vi "position_calculation.vi"(8 "bucket_angle":dbl, 9 "arm_angle":dbl, 10 "boom_angle":dbl) -> (2 "end_point":cluster{"x_axis":dbl, "z_axis":dbl})   [LabVIEW 2020]
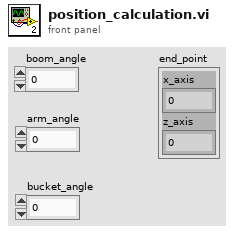
[diagram p1: front panel]
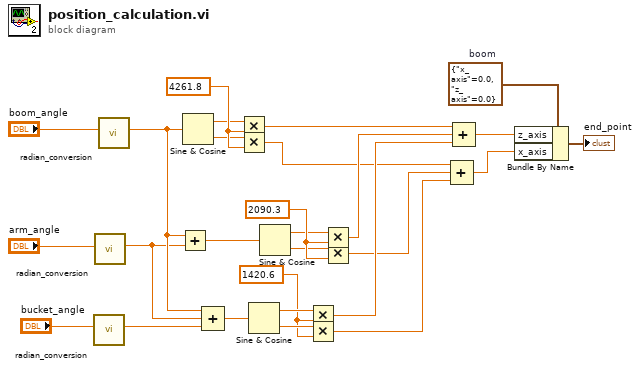
[diagram p0: block diagram]
diagram:
  w18 = cluster{"x_axis":dbl, "z_axis":dbl} {"x_axis"=0.0, "z_axis"=0.0}  # boom
  w25 = 1420.6
  w22 = 4261.8
  w24 = 2090.3
  n1 = call "radian_conversion.vi"("input"="bucket_angle") -> ("output"=w4:dbl)  [unwired: 10 in]
  n2 = call "radian_conversion.vi"("input"="arm_angle") -> ("output"=w5:dbl)  [unwired: 10 in]
  n3 = call "radian_conversion.vi"("input"="boom_angle") -> ("output"=w6:dbl)  [unwired: 10 in]
  n4 = Add(x=w6, y=w5) -> (x+y=w7:dbl)
  n5 = Sine & Cosine(0:w6) -> (1:w21:dbl, 2:w20:dbl)
  n6 = Compound Arithmetic op=ADD(w6, w5, w4) -> (w3:dbl)
  n7 = Multiply(x=w21, y=w22) -> (x*y=w12:dbl)
  n8 = Multiply(x=w20, y=w22) -> (x*y=w8:dbl)
  n9 = Sine & Cosine(0:w3) -> (1:w26:dbl, 2:w27:dbl)
  n10 = Sine & Cosine(0:w7) -> (1:w23:dbl, 2:w19:dbl)
  n11 = Multiply(x=w26, y=w25) -> (x*y=w11:dbl)
  n12 = Multiply(x=w27, y=w25) -> (x*y=w10:dbl)
  n13 = Multiply(x=w23, y=w24) -> (x*y=w13:dbl)
  n14 = Multiply(x=w19, y=w24) -> (x*y=w9:dbl)
  n15 = Compound Arithmetic op=ADD(w8, w9, w10) -> (w1:dbl)
  n16 = Compound Arithmetic op=ADD(w12, w13, w11) -> (w2:dbl)
  n17 = Bundle By Name(cluster=w18, "z_axis"=w2, "x_axis"=w1) -> (→"end_point":cluster{"x_axis":dbl, "z_axis":dbl})
